vi "Read Size.vi"(8 "error in (no error)":errorcluster, 11 "Array in":refnum<class "Vector Parent.lvclass">) -> (0 "error out":errorcluster, 2 "Size":i32, 3 "Array out":refnum<class "Vector Parent.lvclass">)   [LabVIEW 2021, in "Vector Parent.lvclass"]
uses:
  Vector Parent.lvclass
  Vector Parent.lvclass/Vector Parent.ctl
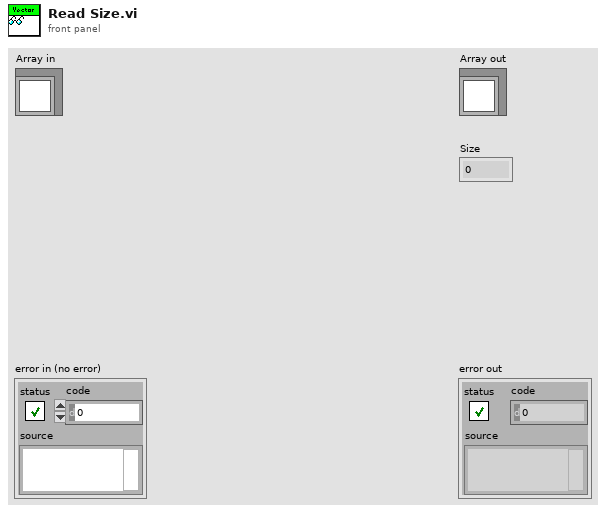
[diagram p1: front panel]
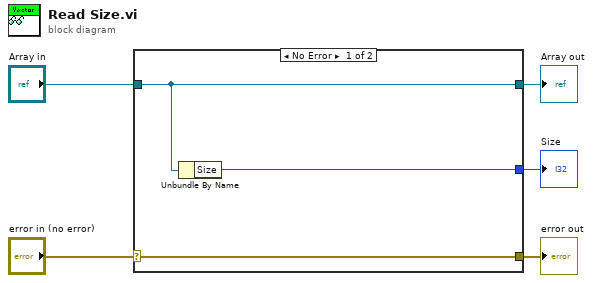
[diagram p0: block diagram]
diagram:
  n1 = case shown="No Error" "error in (no error)" {
    selector: "error in (no error)" -> [w8 w9]
    tunnel: [w8 w9] -> w4
    tunnel: [w7 w10] -> w2
    tunnel: "Array in" -> [w7 w10]
    tunnel: [w6 _] -> w1
    frame No Error {
      n2 = Unbundle By Name(w7) -> ("Size"=w6:u32)
    }
    frame Error {
    }
  }
  "error out" <- w4
  "Array out" <- w2
  "Size" <- w1
